vi "update last messages.vi"(8 "error in (no error)":errorcluster, 11 "Header content in":refnum<class "Header content.lvclass">) -> (0 "error out":errorcluster, 3 "Header content out":refnum<class "Header content.lvclass">)   [LabVIEW 2018, in "Header content.lvclass"]
uses:
  Header content.lvclass
  Header content.lvclass/Header content.ctl
  RxTx/RxTx.lvclass
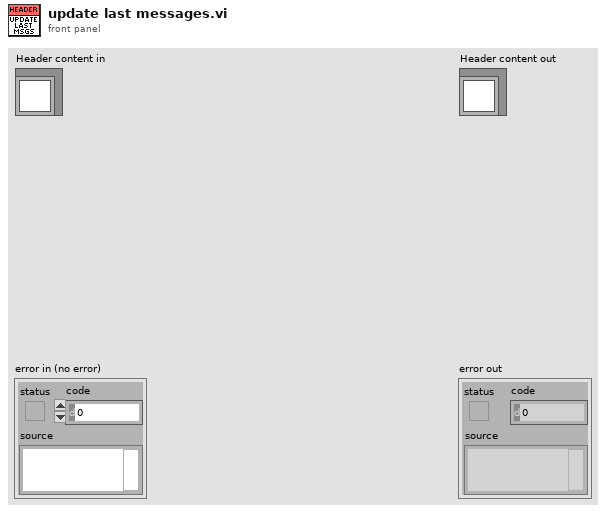
[diagram p1: front panel]
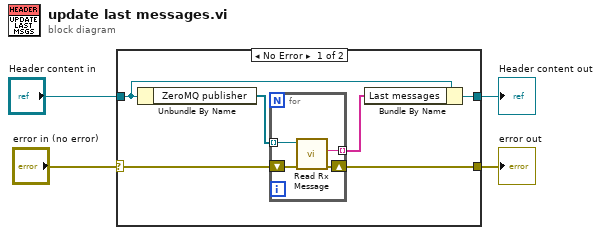
[diagram p0: block diagram]
diagram:
  n1 = case shown="No Error" "error in (no error)" {
    selector: "error in (no error)" -> [w9 w16]
    tunnel: [w8 w16] -> w3
    tunnel: [w6 w15] -> w1
    tunnel: "Header content in" -> [w7 w15]
    frame No Error {
      n2 = Unbundle By Name(w7) -> ("ZeroMQ publisher"=w10:refnum<class "RxTx.lvclass">[])
      n3 = for {
        tunnel: w10 -> [w14] mode=indexing
        tunnel: [w11] -> w5 mode=indexing
        shift-right: [w12] -> w8
        shift-left: w9 -> [w13]
        n4 = call "Read Rx Message.vi"("error in (no error)"=w13, "RxTx in"=w14) -> ("error out"=w12:errorcluster, "Rx Message"=w11:string)  [unwired: 7 in, 1 out]
      }
      n5 = Bundle By Name(cluster=w7, "Last messages"=w5) -> (w6:refnum<class "Header content.lvclass">)
    }
    frame Error {
    }
  }
  "error out" <- w3
  "Header content out" <- w1
